vi "Read State.vi"(8 "error in (no error)":errorcluster, 11 "TCP_Streamer in":refnum<class "TCP_Streamer_Publisher.lvclass">) -> (0 "error out":errorcluster, 2 "State":T1, 3 "TCP_Streamer out":refnum<class "TCP_Streamer_Publisher.lvclass">)   [LabVIEW 2021, in "TCP_Streamer_Publisher.lvclass"]
uses:
  TCP_Streamer_Publisher.lvclass
  Typedef/State.ctl
  TCP_Streamer_Publisher.lvclass/TCP_Streamer_Publisher.ctl
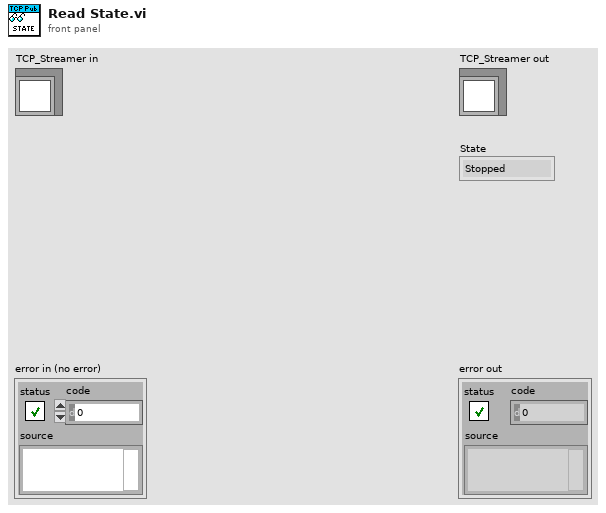
[diagram p1: front panel]
types:
  T1 = typedef "TCP_Streamer_Publisher.lvclass/State.ctl" = enum16{"Stopped", "Listening", "Ready for Data", "Ready to Send", "Sending"}
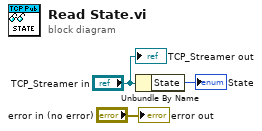
[diagram p0: block diagram]
diagram:
  n1 = Unbundle By Name("TCP_Streamer in") -> ("State"=→"State":T1)
  "error out" <- "error in (no error)"
  "TCP_Streamer out" <- "TCP_Streamer in"
